vi "NI 5783 - Getting Started (Host).vi"() -> ()   [LabVIEW 2017]
uses:
  <vilib>/userdefined/Silver/nirio_resource_slv.ctl
  Program Files (x86)/National Instruments/LabVIEW 2017/examples/FlexRIO/IO Modules/NI 5783/NI 5783 - Getting Started/Controls/Clock Select.ctl
  <vilib>/FPGAPlugInAG/PXIe-7976R/niLvFpga_Open_PXIe-7976R.vi
  <vilib>/rvi/interface/common/dynamic/niFpgaDynamicAddResources.vi
  <vilib>/rvi/interface/common/niFpgaWaitOnOcc.vi
  <vilib>/Utility/error.llb/Error Cluster From Error Code.vi
  <vilib>/rvi/errors/niLvFpgaAdjustHostInterfaceError.vi
  <instrlib>/_niInstr/Streaming/v1/Host/Public/Start Finite Stream.vi
  <instrlib>/_niInstr/Streaming/v1/Host/Public/Wait for Stream.vi
  <vilib>/FPGAPlugInAG/Dynamic/niLvFpga_Close_Dynamic.vi
  <vilib>/rvi/interface/nirviOpenFPGA/nirviOpenFPGA.xnode
  FPGA Bitfiles/ADCSamples_FPGATarget_NI5783-GettingSt_O3Cot-WQFrs.lvbitx
  <vilib>/rvi/interface/nirviMethod/nirviMethod.xnode
  <vilib>/rvi/interface/nirviReadWriteControl/nirviReadWriteControl.xnode
  <vilib>/rvi/interface/nirviCloseFPGA/nirviCloseFPGA.xnode
  <vilib>/rvi/errors/niLvFpgaMergeErrorWithErrorCode.vi
  <instrlib>/_niInstr/Streaming/v1/Host/niInstr Streaming v1 Host.lvlib
  <vilib>/FPGAPlugInAG/Dynamic/niLvFpga_ConfigureFifo_Dynamic.vi
  <vilib>/FPGAPlugInAG/Dynamic/niLvFpga_StartFifo_Dynamic.vi
  NiFpgaLv.dll
  <vilib>/rvi/interface/Simulation/niFpgaSimulationCallBeginRW.vi
  <vilib>/FPGAPlugInAG/Dynamic/niLvFpga_ReadFifo_Dynamic.vi
panel:
  in  "Log File Path":path=path "C:/Users/Admin/Desktop/LIA/ADC Samples/Log Files/test.tdms"
  out "Samples Acquired":i32
  in  "Samples to Acquire":u64=1024
  in  "Trigger Type":enum8{"Immediate", "Data Trigger", "TRIG input"}(ring)
  in  "Clock Select":T1 items=["Internal Clock", "Internal Clock w/ Ref via CLK/REF IN", "Internal Clock w/ Ref via Sync Clock", "External Clock via CLK/REF IN"]
  in  "Rate of External Sample Clock (MHz)":u16=100 min=60 max=100 step=1
  in  "Data Trigger When":enum8{"Trigger Above", "Trigger Below"}(ring)
  out "AI":waveform(dbl)[](graph)
  out "Error Out":errorcluster
  in  "Data Trigger Level (V)":dbl
  in  "stop":bool
  in  "Record Size":u64=1024
  in  "RIO Resource":T2="RIO0"
  # "Resource Configuration"
  # "AI Configuration"
  # "Ignored when Internal Clock is selected"
  # "AI Configuration"
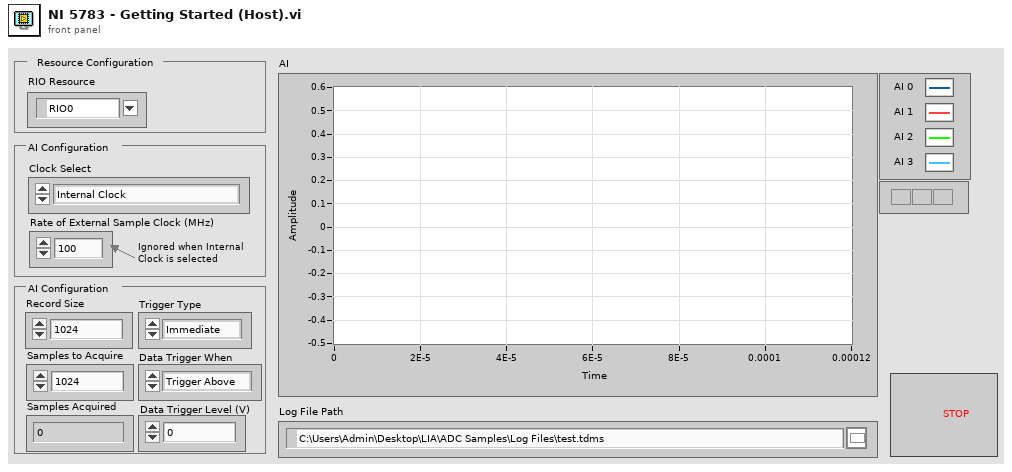
[diagram p1: front panel]
types:
  T1 = typedef "Clock Select.ctl" = u16
  T2 = typedef "nirio_resource_slv.ctl" = tag
  T3 = enum16{"open", "open or create", "create or replace", "create", "open (read-only)"}
  T4 = cluster{"level":i16, "trigger when":enum8{"Trigger Above", "Trigger Below"}}
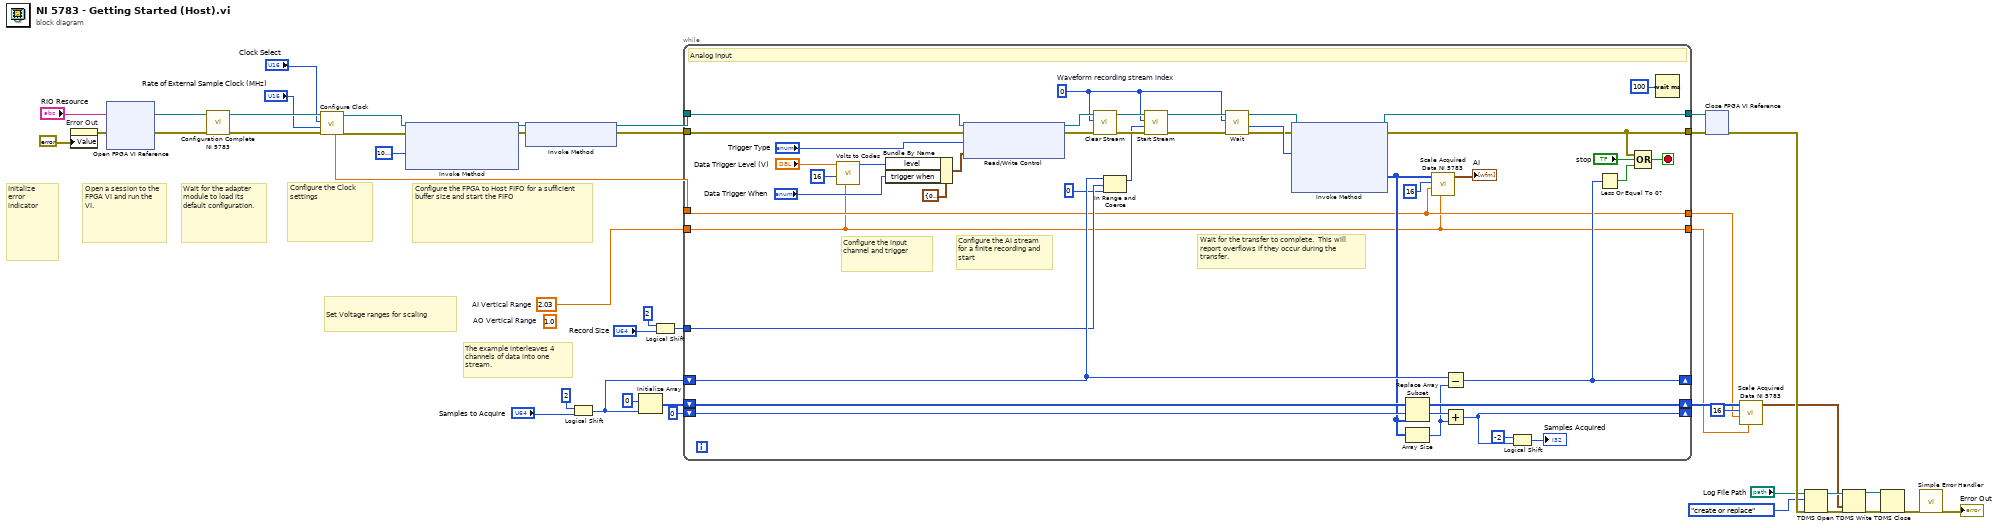
[diagram p0: block diagram]
diagram:
  w33 = 2.03  # AI Vertical Range
  (unwired) 1.0  # AO Vertical Range
  # "The example interleaves 4 channels of data into one stream."
  # "Configure the Clock settings"
  # "Configure the FPGA to Host FIFO for a sufficient buffer size and start the FIFO"
  # "Wait for the adapter module to load its default configuration."
  # "Open a session to the FPGA VI and run the VI."
  # "Set Voltage ranges for scaling"
  # "Initalize error indicator"
  n1 = property on="Error Out" class="Clust (strict)"("Value"=errorcluster {"status"=FALSE, "code"=0, "source"=""} ("error out")) -> (error out=w41:errorcluster)  [unwired: 2 in, 1 out]
  n2 = xnode "Open FPGA VI Reference"("error in"=w41, "resource name"="RIO Resource") -> ("FPGA VI Reference Out"=w32:refnum<k20>, "error out"=w31:errorcluster)
  n3 = call "Configuration Complete NI 5783.vi"("error in"=w31, "FPGA VI Reference In"=w32) -> ("error out"=w29:errorcluster, "FPGA VI Reference Out"=w30:refnum<k20>)  [unwired: 7 in, 1 out]
  n4 = call "Configure Clock.vi"("error in (no error)"=w29, "Rate of External Sample Clock (MHz)"="Rate of External Sample Clock (MHz)", "Clock Select"="Clock Select", "FPGA VI Reference In"=w30) -> ("error out"=w27:errorcluster, "FPGA VI Reference Out"=w28:refnum<k20>, "Sampling Rate"=w24:dbl)  [unwired: 3 in, 2 out]
  n5 = xnode "Invoke Method"("FPGA VI Reference In"=w28, "error in"=w27, "Requested Depth"=u32 1024000) -> ("FPGA VI Reference Out"=w37:refnum<k20>, "error out"=w36:errorcluster)  [unwired: 1 out]
  n6 = xnode "Invoke Method"("FPGA VI Reference In"=w37, "error in"=w36) -> ("FPGA VI Reference Out"=w39:refnum<k20>, "error out"=w38:errorcluster)
  n7 = Logical Shift(y=u16 2, x="Samples to Acquire") -> (x << y=w17:u64)
  n8 = Initialize Array(i16 0 ("element"), w17) -> (w21:i16[])
  n9 = Logical Shift(y=u16 2, x="Record Size") -> (x << y=w14:u64)
  n10 = while {
    tunnel: [w84] -> w43
    tunnel: w39 -> [w83]
    tunnel: w33 -> [w49]
    tunnel: w38 -> [w82]
    tunnel: [w71] -> w23
    tunnel: w24 -> [w50]
    shift-right: [w59] -> _
    shift-left: w17 -> [w54]
    shift-right: [w56] -> w12
    shift-left: w21 -> [w57]
    shift-right: [w48] -> _
    shift-left: 0 ("index") -> [w55]
    tunnel: w14 -> [w53]
    tunnel: [w50] -> w10
    tunnel: [w49] -> w11
    stop <- w60 stop-if-true
    w61 = 0  # Waveform recording stream index
    # "Wait for the transfer to complete.  This will report overflows if they occur during the transfer."
    # "Configure the AI stream for a finite recording and start"
    # "Configure the input channel and trigger"
    # "Analog Input"
    n11 = call "Volts to Codes.vi"("range (Vpp)"=w49, "Number of Bits"=i16 16, "Volts In"="Data Trigger Level (V)") -> ("ADC Codes Out"=w67:i16)  [unwired: 8 in]
    n12 = Bundle By Name(cluster=T4 {"level"=0, "trigger when"=enum."Trigger Above"} ("Trigger Configuration"), "level"=w67, "trigger when"="Data Trigger When") -> (w70:T4)
    n13 = xnode "Read/Write Control"("FPGA VI Reference In"=w83, "error in"=w82, "Trigger Type"="Trigger Type", "Trigger Configuration"=w70) -> ("FPGA VI Reference Out"=w65:refnum<k20>, "error out"=w64:errorcluster)
    n14 = call <instrlib>:"Clear Stream.vi"("error in (no error)"=w64, "stream index"=w61, "refnum in"=w65) -> ("error out"=w63:errorcluster, "refnum out"=w62:refnum<k20>)  [unwired: 7 in]
    n15 = In Range and Coerce(upper limit=w54, x=w53, lower limit=u64 0) -> (coerced(x)=w44:u64)  [unwired: 1 out]
    n16 = call-poly <instrlib>:"Start Stream.vi"("error in (no error)"=w63, "num samples"=w44, "stream index"=w61, "refnum in"=w62) -> ("error out"=w76:errorcluster, "refnum out"=w74:refnum<k20>)  [unwired: 6 in]
    n17 = call-poly <instrlib>:"Wait.vi"("error in (no error)"=w76, "stream index"=w61, "refnum in"=w74) -> ("error out"=w72:errorcluster, "samples transferred"=w75:u64, "refnum out"=w73:refnum<k20>)  [unwired: 5 in, 1 out]
    n18 = xnode "Invoke Method"("FPGA VI Reference In"=w73, "error in"=w72, "Number of Elements"=w75) -> ("FPGA VI Reference Out"=w84:refnum<k20>, "error out"=w71:errorcluster, "Data"=w51:i16[])  [unwired: 1 in, 1 out]
    n19 = Replace Array Subset(array=w57, new element=w51, index=w55) -> (w56:i16[])
    n20 = Array Size(array=w51) -> (size(s)=w52:i32)
    n21 = call "Scale Acquired Data NI 5783.vi"("range (V)"=w49, "Sample Rate"=w50, "Number of Bits"=i16 16, "Data In"=w51) -> ("Data"=→"AI":waveform(dbl)[])  [unwired: 7 in]
    n22 = Subtract(x=w54, y=w52) -> (x-y=w59:u64)
    n23 = Add(x=w55, y=w52) -> (x+y=w48:i32)
    n24 = Logical Shift(y=i16 -2, x=w48) -> (x << y=→"Samples Acquired":i32)
    n25 = Less Or Equal To 0?(x=w59) -> (x <= 0?=w58:bool)
    n26 = Compound Arithmetic op=OR(w71, "stop", w58) -> (w60:bool)
    n27 = Wait (ms)(milliseconds to wait=u32 100) -> ()  [unwired: 1 out]
  }
  n28 = xnode "Close FPGA VI Reference"("FPGA VI Reference In"=w43, "error in"=w23) -> ("error out"=w9:errorcluster)
  n29 = call "Scale Acquired Data NI 5783.vi"("range (V)"=w11, "Sample Rate"=w10, "Number of Bits"=i16 16, "Data In"=w12) -> ("Data"=w5:waveform(dbl)[])  [unwired: 7 in]
  n30 = TDMS Open(8:w9, 10:T3."create or replace" ("operation (0:open)"), 11:"Log File Path") -> (0:w6:errorcluster, 3:w7:refnum<k34>)  [unwired: 4 in]
  n31 = TDMS Write(0:w7, 9:w5, 11:w6) -> (4:w4:refnum<k34>, 15:w3:errorcluster)  [unwired: 3 in, 2 out]
  n32 = TDMS Close(8:w3, 11:w4) -> (0:w2:errorcluster)  [unwired: 1 out]
  n33 = call <vilib>:"Simple Error Handler.vi"("error in (no error)"=w2) -> ("error out"=→"Error Out":errorcluster)  [unwired: 4 in, 4 out]
